vi "PIDTEMPtest6.vi"() -> ()   [LabVIEW 2015]
uses:
  <vilib>/DAQmx/write.llb/DAQmx Write (Digital 1D Bool NChan 1Samp 1Line).vi
  <vilib>/DAQmx/write.llb/DAQmx Write (Digital Bool 1Line 1Point).vi
  <vilib>/DAQmx/read.llb/DAQmx Read (Analog DBL 1Chan 1Samp).vi
  <vilib>/DAQmx/miscellaneous.llb/DAQmx Fill In Error Info.vi
  <vilib>/addons/control/pid/NI_PID_autopid.lvlib
panel:
  in  "Heater On/Off":bool
  in  "Manual Control":bool
  out "ms to wait":dbl
  out "Control Value":dbl
  in  "setpoint in C":dbl format="%.2f"
  in  "reinitialize? (F)":bool
  in  "autotune? (F)":bool
  out "PID gains out":T1={"proportional gain (Kc)"=1.0, "integral time (Ti, min)"=0.01, "derivative time (Td, min)"=0.0} {"derivative time (Td, min)" format="%.3f"; "integral time (Ti, min)" format="%.3f"; "proportional gain (Kc)" format="%.3f"}
  in  "PID gains":T1={"proportional gain (Kc)"=1.0, "integral time (Ti, min)"=0.01, "derivative time (Td, min)"=0.0} {"derivative time (Td, min)" format="%.3f"; "integral time (Ti, min)" format="%.3f"; "proportional gain (Kc)" format="%.3f"}
  in  "autotuning parameters":T2={"controller type"=1, "relay cycles"=3, "relay amplitude"=1.0, "control specification"=2, "PV noise level"=0.1} {"PV noise level" format="%.2f"; "control specification" items=["normal", "fast", "slow"]; "relay amplitude" format="%.2f"; "controller type" items=["PID", "PI", "P"]}
  in  "stop":bool
  out "Temp":dbl
  out "Temp Chart 2":dbl(graph)
  out "Temp Chart":dbl(graph)
  out "Temp(C)":dbl(slide) scale=-10.0..100.0
  out "Temperature (Celcius)":dbl format="%#.1g"
  out "Voltage Reading(Temp)":dbl format="%#_13g"
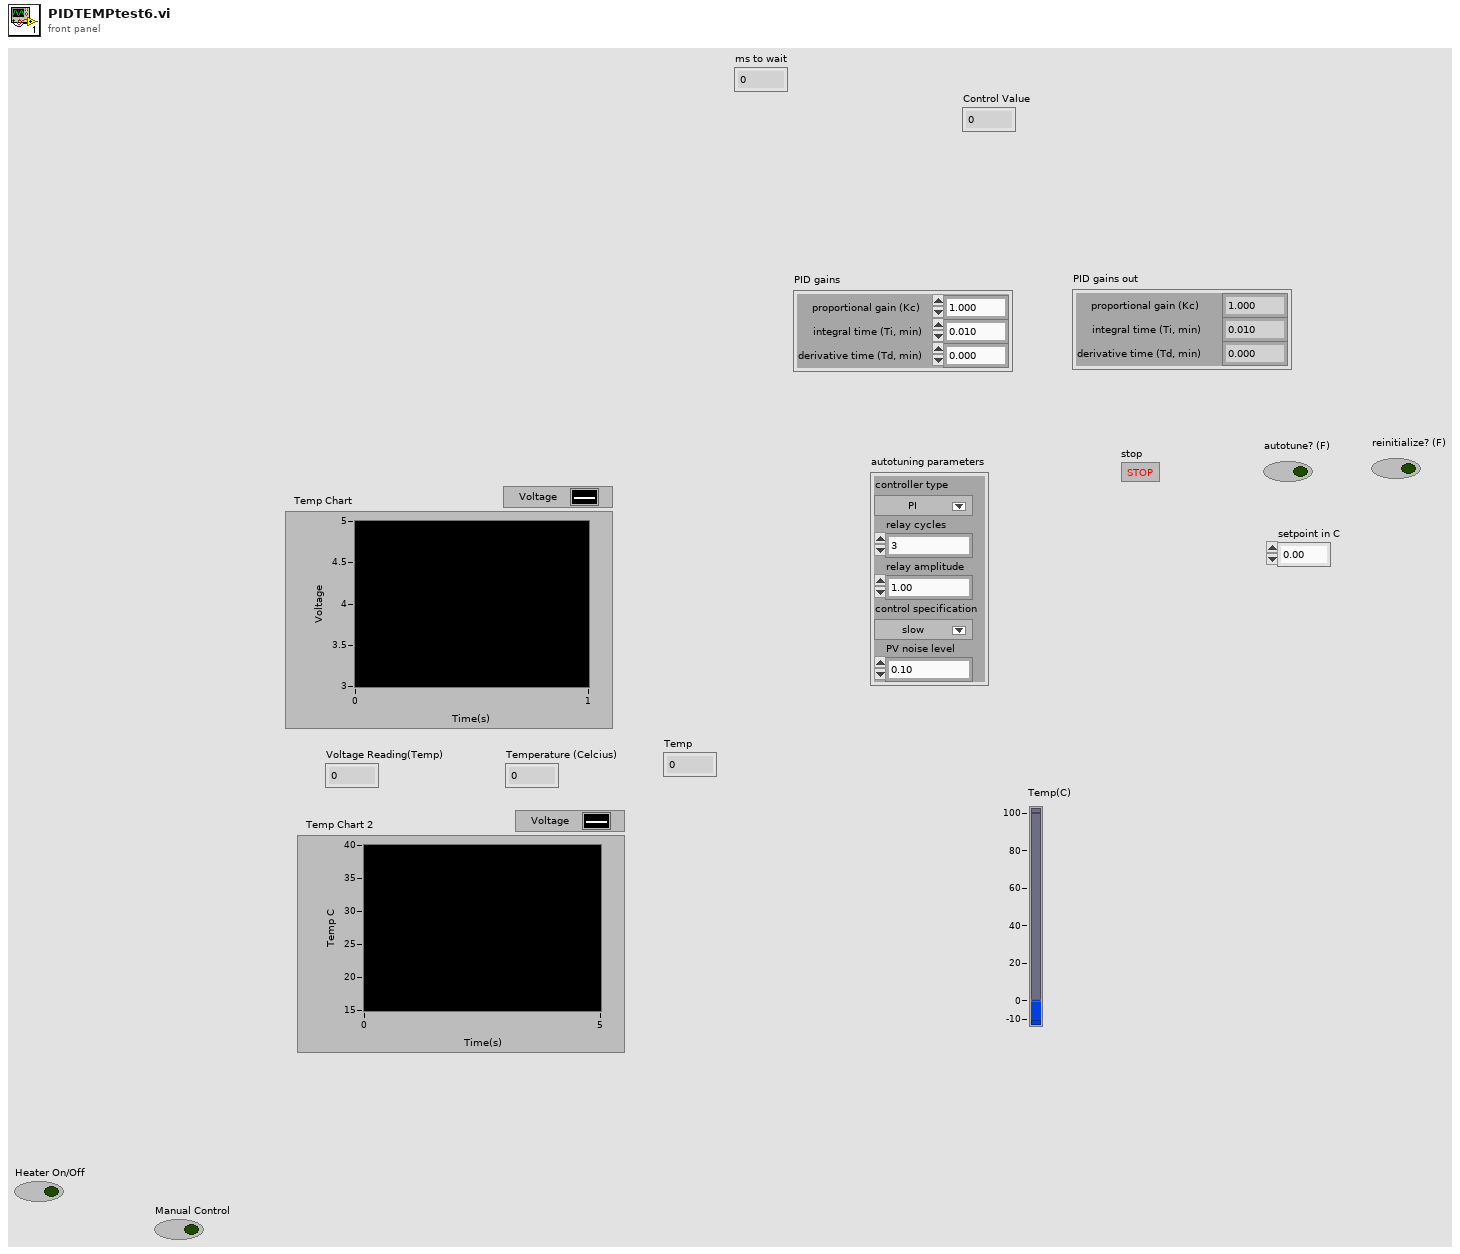
[diagram p1: front panel]
types:
  T1 = cluster{"proportional gain (Kc)":dbl, "integral time (Ti, min)":dbl, "derivative time (Td, min)":dbl}
  T2 = cluster{"controller type":u16, "relay cycles":i32, "relay amplitude":dbl, "control specification":u16, "PV noise level":dbl}
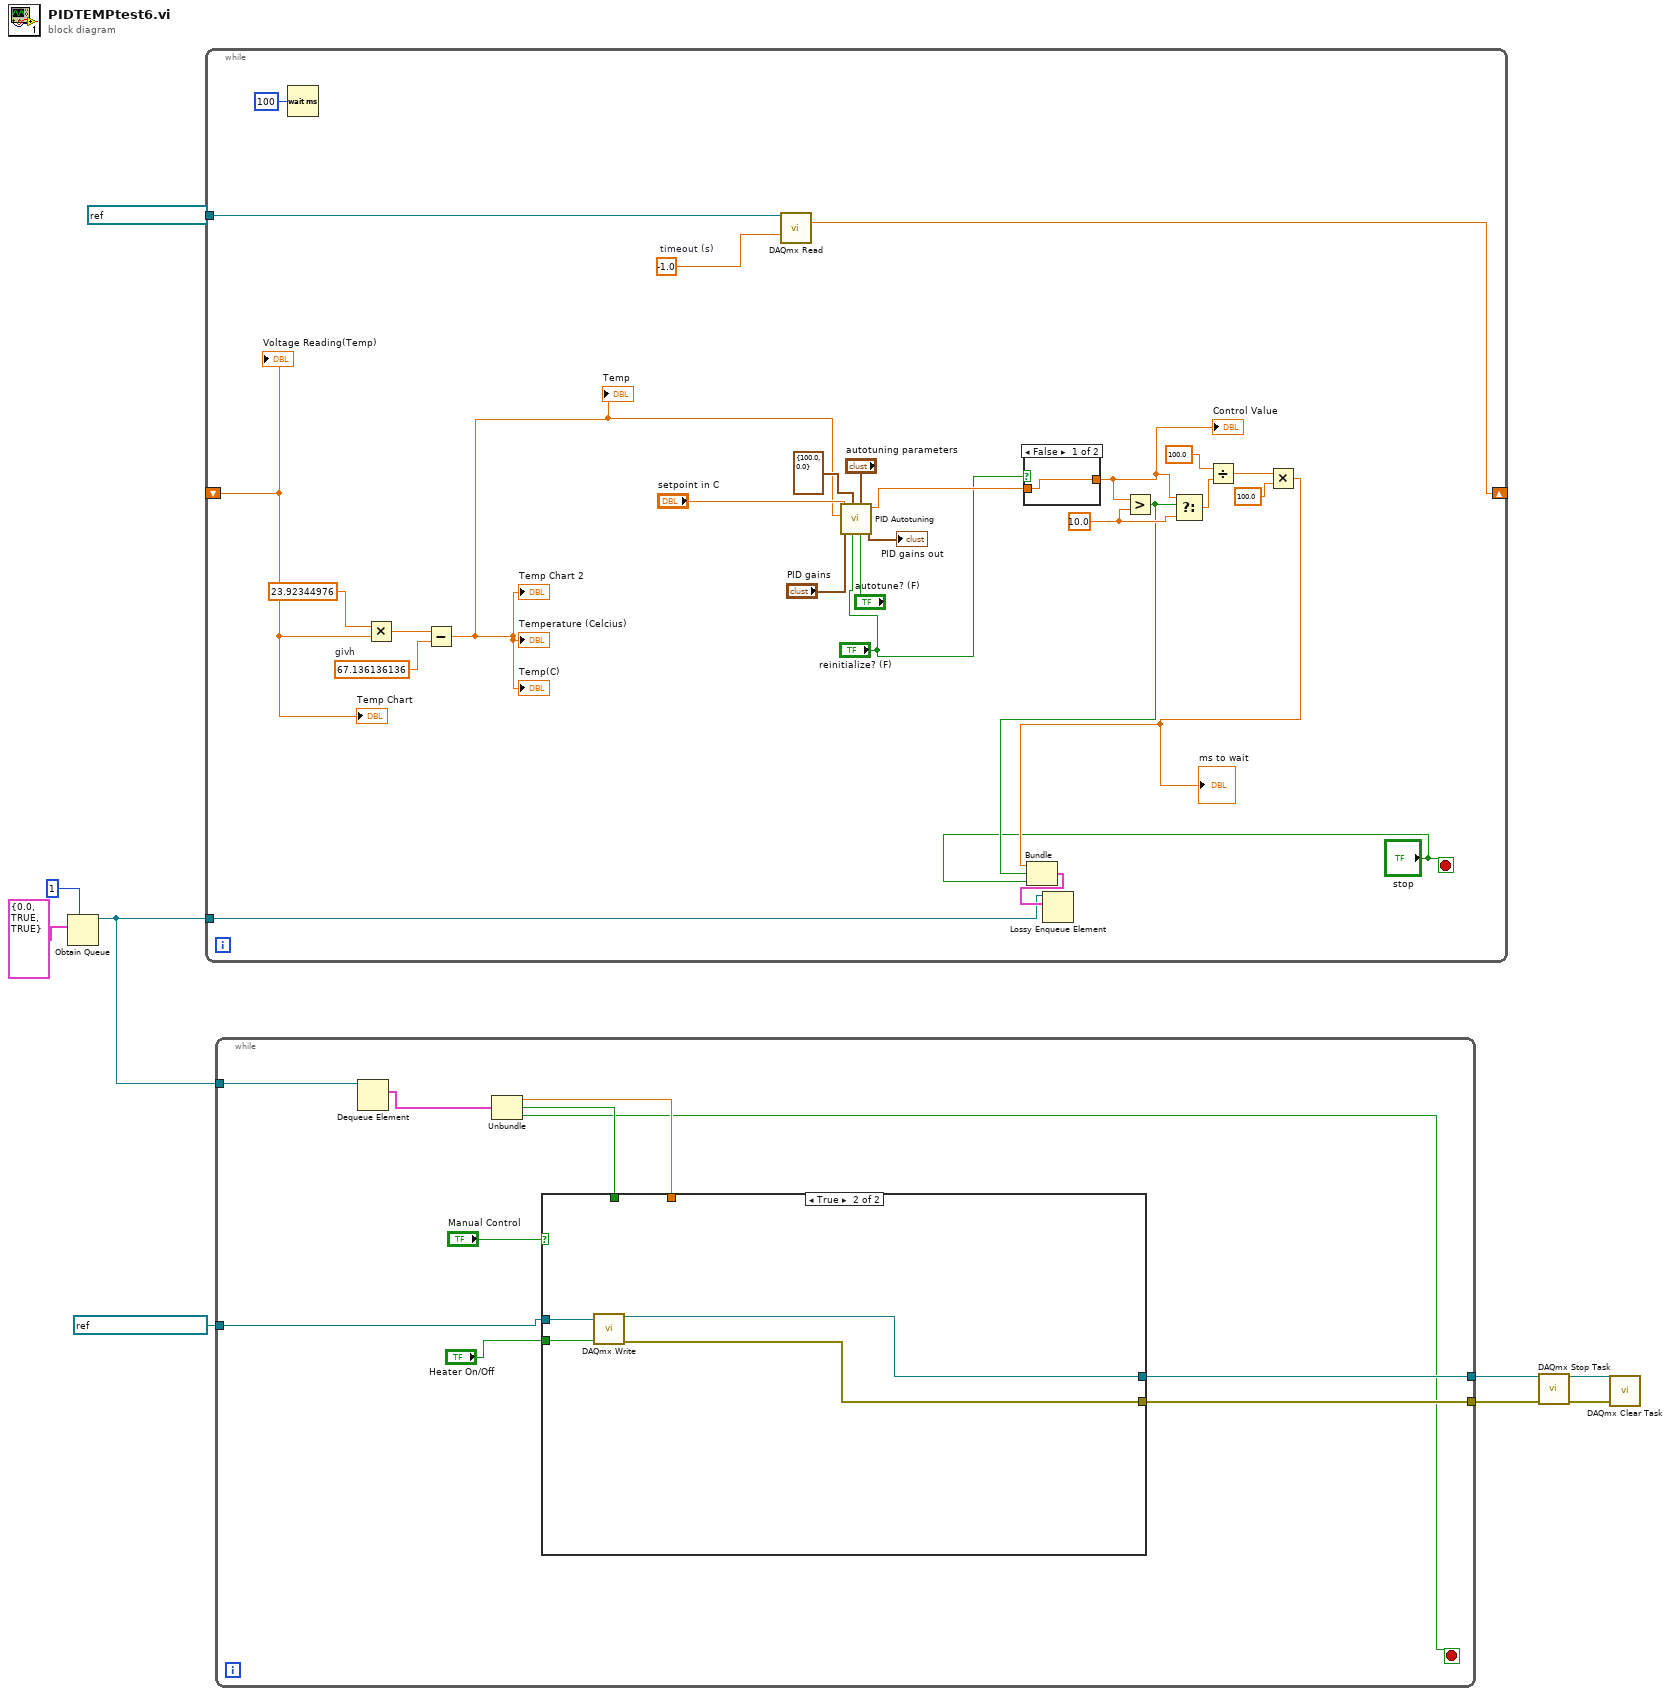
[diagram p0: block diagram]
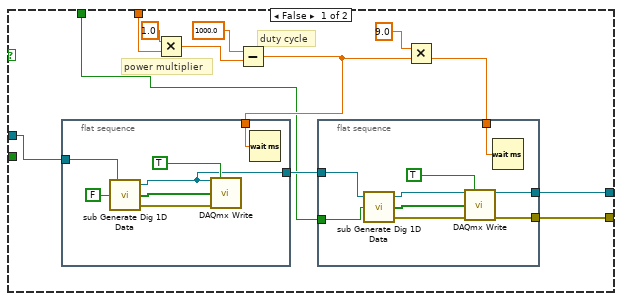
[diagram p2: hidden frame]
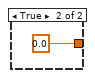
[diagram p3: hidden frame]
diagram:
  n1 = Obtain Queue(max queue size (-1, unlimited)=1, element data type=cluster{dbl, bool, bool} {0.0, TRUE, TRUE}) -> (queue out=w7:refnum<queue>)  [unwired: 3 in, 2 out]
  n2 = while {
    tunnel: refnum<k21> "MyVoltageTask_0" -> [w33]
    shift-right: [w16] -> _
    shift-left: _ -> [w17]
    tunnel: w7 -> [w11]
    stop <- "stop" stop-if-true
    w19 = 10.0 ("f")
    w34 = 67.136136136  # givh
    w37 = -1.0  # timeout (s)
    n3 = Wait (ms)(milliseconds to wait=u32 100) -> ()  [unwired: 1 out]
    n4 = Multiply(x=23.92344976, y=w17) -> (x*y=w35:dbl)
    n5 = Subtract(x=w35, y=w34) -> (x-y=w15:dbl)
    "Temperature (Celcius)" <- w15
    "Temp(C)" <- w15
    "Temp Chart 2" <- w15
    "Temp" <- w15
    n6 = call-poly <vilib>:"DAQmx Read.vi"("task/channels in"=w33, "timeout"=w37) -> ("data"=w16:dbl)  [unwired: 11 in, 2 out]
    n7 = call <vilib>:"PID Autotuning.vi"("autotune? (F)"="autotune? (F)", "autotuning parameters"="autotuning parameters", "reinitialize? (F)"="reinitialize? (F)", "output range"=cluster{"output high":dbl, "output low":dbl} {"output high"=100.0, "output low"=0.0}, "PID gains"="PID gains", "process variable"=w15, "setpoint"="setpoint in C") -> ("PID gains out"=→"PID gains out":T1, "output"=w27:dbl)  [unwired: 1 in, 2 out]
    n8 = case shown="False" "reinitialize? (F)" {
      tunnel: [w38 0.0] -> w20
      tunnel: w27 -> [w38 _]
      frame False {
      }
      frame True {
      }
    }
    "Control Value" <- w20
    n9 = Greater?(x=w20, y=w19) -> (0:w13:bool)
    n10 = Select(t=w20, s=w13, f=w19) -> (s? t:f=w21:dbl)
    n11 = Divide(x=100.0, y=w21) -> (x/y=w23:dbl)
    n12 = Multiply(x=w23, y=100.0) -> (x*y=w14:dbl)
    "ms to wait" <- w14
    n13 = Bundle(w14, w13, "stop"="stop") -> (w12:cluster{dbl, bool, "stop":bool})  [unwired: 1 in]
    n14 = Lossy Enqueue Element(queue=w11, element=w12) -> ()  [unwired: 1 in, 4 out]
    "Voltage Reading(Temp)" <- w17
    "Temp Chart" <- w17
  }
  n15 = while {
    tunnel: w7 -> [w49]
    tunnel: refnum<k21> "MyDigitalOutTask_2" -> [w46]
    tunnel: [w42] -> w4
    tunnel: [w41] -> w3
    stop <- w40 stop-if-true
    n16 = Dequeue Element(queue=w49) -> (element=w45:cluster{dbl, bool, bool})  [unwired: 2 in, 3 out]
    n17 = Unbundle(w45) -> (w44:dbl, w43:bool, w40:bool)
    n18 = case shown="True" "Manual Control" {
      tunnel: w46 -> [w60 w81]
      tunnel: "Heater On/Off" -> [_ w80]
      tunnel: w44 -> [w59 _]
      tunnel: w43 -> [w54 _]
      tunnel: [w51 w79] -> w42
      tunnel: [w50 w78] -> w41
      frame False {
        # "duty cycle"
        # "power multiplier"
        n19 = flat-sequence {
          tunnel: w60 -> [w74]
          tunnel: [w73] -> w61
          tunnel: w58 -> [w72]
          frame #0 {
            n20 = call <vilib>:"sub Generate Dig 1D Data.vi"("initial value"=FALSE, "task in"=w74) -> ("error out"=w76:errorcluster, "Data"=w77:bool[], "task out"=w73:refnum<k21>)  [unwired: 1 in]
            n21 = call-poly <vilib>:"DAQmx Write.vi"("task/channels in"=w73, "auto start"=TRUE, "data"=w77, "error in"=w76) -> ()  [unwired: 9 in, 3 out]
            n22 = Wait (ms)(milliseconds to wait=w72) -> ()  [unwired: 1 out]
          }
        }
        n23 = Multiply(x=1.0, y=w59) -> (x*y=w53:dbl)
        n24 = Subtract(x=1000.0, y=w53) -> (x-y=w58:dbl)
        n25 = flat-sequence {
          tunnel: w61 -> [w66]
          tunnel: w56 -> [w65]
          tunnel: w54 -> [w64]
          tunnel: [w63] -> w51
          tunnel: [w62] -> w50
          frame #0 {
            n26 = call <vilib>:"sub Generate Dig 1D Data.vi"("initial value"=w64, "task in"=w66) -> ("error out"=w69:errorcluster, "Data"=w67:bool[], "task out"=w68:refnum<k21>)  [unwired: 1 in]
            n27 = call-poly <vilib>:"DAQmx Write.vi"("task/channels in"=w68, "auto start"=TRUE, "data"=w67, "error in"=w69) -> ("task out"=w63:refnum<k21>, "error out"=w62:errorcluster)  [unwired: 9 in, 1 out]
            n28 = Wait (ms)(milliseconds to wait=w65) -> ()  [unwired: 1 out]
          }
        }
        n29 = Multiply(x=9.0, y=w58) -> (x*y=w56:dbl)
      }
      frame True {
        n30 = call-poly <vilib>:"DAQmx Write.vi"("task/channels in"=w81, "data"=w80) -> ("task out"=w79:refnum<k21>, "error out"=w78:errorcluster)  [unwired: 11 in, 1 out]
      }
    }
  }
  n31 = call <vilib>:"DAQmx Stop Task.vi"("task/channels in"=w4, "error in"=w3) -> ("task out"=w2:refnum<k21>, "error out"=w1:errorcluster)  [unwired: 12 in]
  n32 = call <vilib>:"DAQmx Clear Task.vi"("task in"=w2, "error in"=w1) -> ()  [unwired: 13 in, 1 out]
